vi "HeatingExperiment_7_ForLoops.vi"() -> ()   [LabVIEW 2017]
uses:
  <vilib>/DAQmx/read.llb/DAQmx Read (Analog 1D DBL NChan 1Samp).vi
  <vilib>/DAQmx/create/channels.llb/DAQmx Create Channel (AI-Voltage-Basic).vi
  <vilib>/DAQmx/miscellaneous.llb/DAQmx Fill In Error Info.vi
  <vilib>/Utility/file.llb/Write Delimited Spreadsheet (DBL).vi
panel:
  in  "manual Temp. ?":bool=TRUE
  in  "Step Vdc (v)":i32=5
  in  "Starting Vdc (v)":dbl=10.0 format="%#_13g"
  out "data":dbl[](array[numeric]) format="%0.2f"
  in  "Manual Voltage (V)":dbl
  out "Loop 2":i32
  out "Loop out":i32
  out "Time 2":dbl
  out "Time 1":dbl
  out "Time":dbl
  out "No. of  loops (Heater OFF)":dbl
  out "No. of  loops (Heater On)":dbl
  out "No. of loops ON + OFF":dbl
  out "Temperature (C)":dbl[](array[numeric])
  out "Waveform Chart":cluster{dbl, dbl}(graph)
  in  "folder path":path
  in  "Stop Temperature Acquisition":bool
  out "thermocouples (V)":dbl[](array[numeric]) format="%0.4f"
  out "Vdc measured":dbl format="%.2p"
  out "Idc measured":dbl format="%.2p"
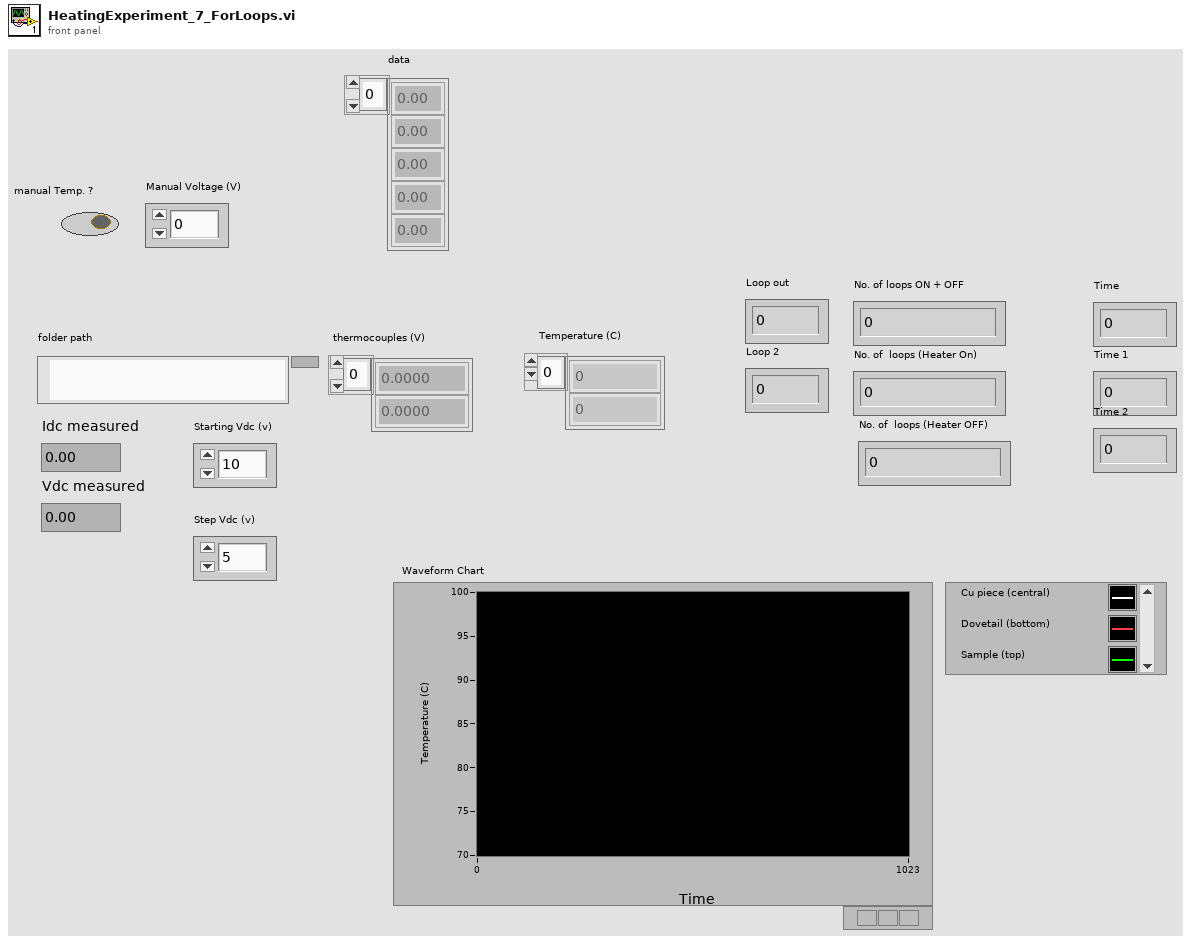
[diagram p1: front panel]
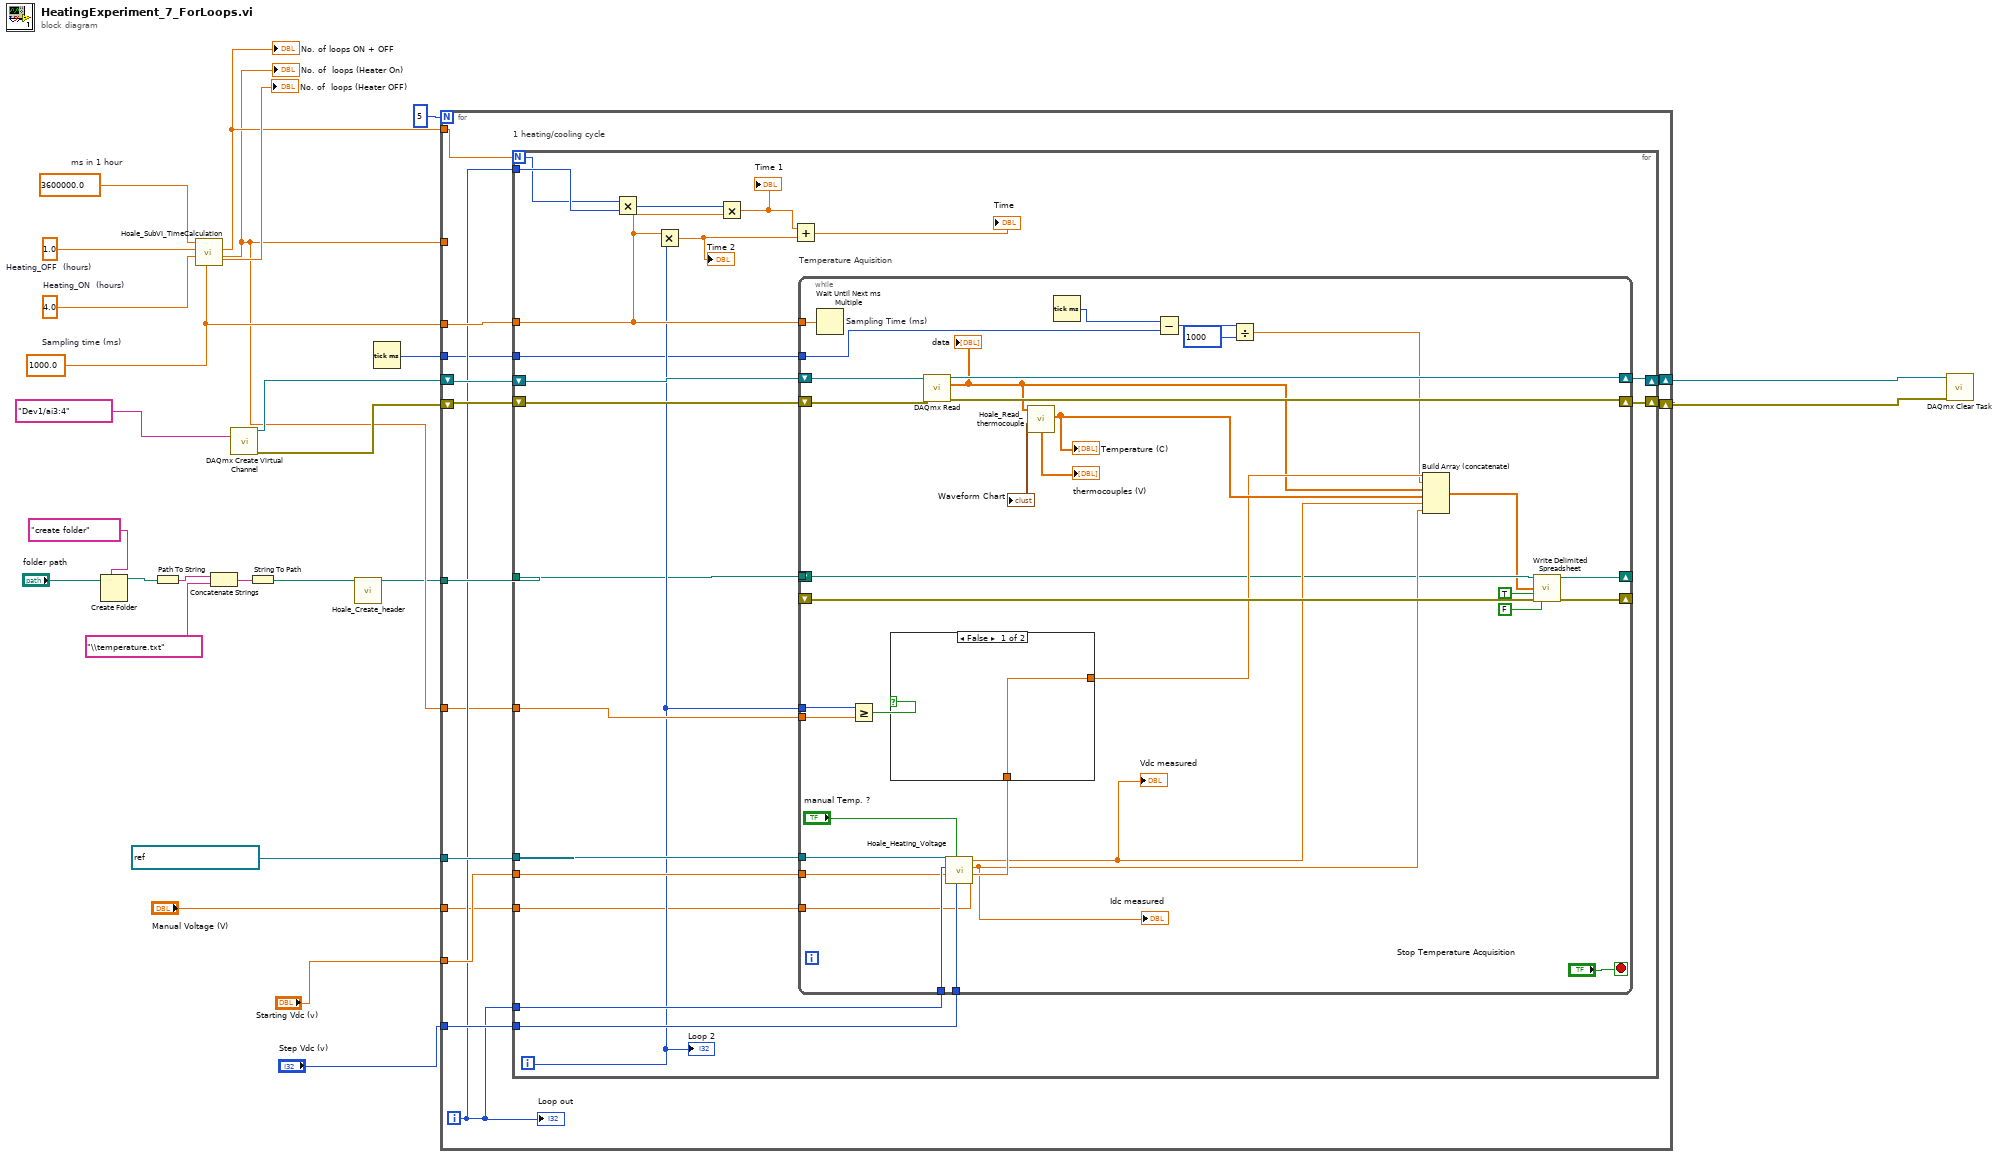
[diagram p0: block diagram]
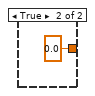
[diagram p2: hidden frame]
diagram:
  w10 = 1.0  # Heating_OFF  (hours)
  w8 = 3600000.0  # ms in 1 hour
  w9 = 1000.0  # Sampling time (ms)
  w11 = 4.0  # Heating_ON  (hours)
  n1 = Create Folder(prompt (Create Folder)="create folder", path (use dialog)="folder path") -> (created path=w17:path)  [unwired: 1 in, 2 out]
  n2 = Path To String(path=w17) -> (string=w22:string)
  n3 = call "Hoale_SubVI_TimeCalculation.vi"("Sampling time (ms)"=w9, "Heating_ON  (hours)"=w11, "Heating_OFF  (hours)"=w10, "No. of ms in 1 hour"=w8) -> ("No. of  loops (Heater On)"=w5:dbl, "No. of loops ON + OFF"=w6:dbl, "No. of  loops (Heater OFF)"=→"No. of  loops (Heater OFF)":dbl)  [unwired: 2 in, 3 out]
  "No. of loops ON + OFF" <- w6
  "No. of  loops (Heater On)" <- w5
  n4 = Concatenate Strings(w22, "\\temperature.txt") -> (w20:string)
  n5 = call-poly <vilib>:"DAQmx Create Virtual Channel.vi"("physical channels"=tag "Dev1/ai3:4") -> ("task out"=w25:refnum<k21>, "error out"=w24:errorcluster)  [unwired: 13 in]
  n6 = String To Path(string=w20) -> (path=w3:path)
  n7 = call "Hoale_Create_header.vi"("File Path Control"=w3) -> ("path"=w2:path)  [unwired: 9 in, 1 out]
  n8 = Tick Count (ms)() -> (millisecond timer value=w1:u32)
  n9 = for {
    N: 5 -> [_]
    tunnel: w2 -> [w38]
    shift-right: [w32] -> w13
    shift-left: w25 -> [w40]
    shift-right: [w33] -> w12
    shift-left: w24 -> [w39]
    tunnel: w9 -> [w37]
    tunnel: "Step Vdc (v)" -> [w34]
    tunnel: "Starting Vdc (v)" -> [w35]
    tunnel: refnum<k15> "GPIB8::5::INSTR" ("resource name (\"GPIB::14::INSTR\")") -> [w36]
    tunnel: w6 -> [w31]
    tunnel: w5 -> [_]
    tunnel: w5 -> [w29]
    tunnel: "Manual Voltage (V)" -> [w28]
    tunnel: w1 -> [w27]
    i -> [w30]
    n10 = for "1 heating/cooling cycle" {
      N: w31 -> [w51]
      tunnel: w38 -> [w42]
      tunnel: w37 -> [w46]
      tunnel: w36 -> [w58]
      tunnel: w35 -> [w57]
      tunnel: w34 -> [w56]
      tunnel: w30 -> [w55]
      shift-right: [w54] -> w32
      shift-left: w40 -> [w60]
      shift-right: [w53] -> w33
      shift-left: w39 -> [w59]
      tunnel: w30 -> [w52]
      tunnel: w29 -> [w45]
      tunnel: w28 -> [w43]
      tunnel: w27 -> [w41]
      i -> [w44]
      n11 = Multiply(x=w51, y=w52) -> (x*y=w49:i32)
      n12 = Multiply(x=w46, y=w44) -> (x*y=w50:dbl)
      "Time 2" <- w50
      n13 = Multiply(x=w49, y=w46) -> (x*y=w48:dbl)
      "Time 1" <- w48
      n14 = Add(x=w48, y=w50) -> (x+y=→"Time":dbl)
      n15 = while "Temperature Aquisition" {
        shift-right: [w91] -> w54
        shift-left: w60 -> [w95]
        shift-right: [w93] -> w53
        shift-left: w59 -> [w94]
        shift-right: [w74] -> _
        shift-left: _ -> [w73]
        shift-right: [w75] -> _
        shift-left: _ -> [_]
        tunnel: w46 -> [w90]
        tunnel: w58 -> [w87]
        tunnel: w55 -> [w85]
        tunnel: w57 -> [w84]
        tunnel: w56 -> [w83]
        tunnel: w45 -> [w81]
        tunnel: w44 -> [w80]
        tunnel: w43 -> [w79]
        tunnel: w42 -> [w67]
        tunnel: w41 -> [w64]
        stop <- "Stop Temperature Acquisition" stop-if-true
        n16 = Wait Until Next ms Multiple "Sampling Time (ms)"(millisecond multiple=w90) -> ()  [unwired: 1 out]
        n17 = Greater Or Equal?(x=w80, y=w81) -> (x >= y?=w92:bool)
        n18 = call-poly <vilib>:"DAQmx Read.vi"("task/channels in"=w95, "error in"=w94) -> ("task out"=w91:refnum<k21>, "data"=w68:dbl[], "error out"=w93:errorcluster)  [unwired: 11 in]
        "data" <- w68
        n19 = call "Hoale_Heating_Voltage.vi"("Manual Voltage (V)"=w79, "step Vdc (v)"=w83, "manual Temp. ?"="manual Temp. ?", "Starting Vdc (v)"=w84, "Number of loops"=w85, "GPIB input"=w87) -> ("Set Voltage"=w86:dbl, "Measured Current"=w72:dbl, "Measured Voltage"=w71:dbl)  [unwired: 3 in]
        "Idc measured" <- w72
        "Vdc measured" <- w71
        n20 = case shown="False" w92 {
          tunnel: [w96 0.0 ("Voltage Level (0.0)")] -> w69
          tunnel: w86 -> [w96 _]
          frame False {
          }
          frame True {
          }
        }
        n21 = call "Hoale_Read_thermocouple.vi"("data"=w68) -> ("Cluster"=→"Waveform Chart":cluster{"th1":cdb, "th0":cdb}, "Temp. Array"=w70:cdb[], "thermocouples (V)"=→"thermocouples (V)":dbl[])  [unwired: 8 in]
        "Temperature (C)" <- w70
        n22 = Tick Count (ms)() -> (millisecond timer value=w65:u32)
        n23 = Subtract(x=w65, y=w64) -> (x-y=w63:u32)
        n24 = Divide(x=w63, y=u32 1000) -> (x/y=w61:dbl)
        n25 = Build Array (concatenate) "Build Array"(w69, w61, w68, w70, w71, w72) -> (w66:cdb[])
        n26 = call-poly <vilib>:"Write Delimited Spreadsheet.vi"("file path (dialog if empty)"=w67, "1D data"=w66, "append to file? (new file:F)"=TRUE, "error in (no error)"=w73, "transpose? (no:F)"=FALSE) -> ("new file path (Not A Path if cancelled)"=w75:path, "error out"=w74:errorcluster)  [unwired: 9 in]
      }
      "Loop 2" <- w44
    }
    "Loop out" <- w30
  }
  n27 = call <vilib>:"DAQmx Clear Task.vi"("task in"=w13, "error in"=w12) -> ()  [unwired: 13 in, 1 out]
